vi "Main.vi"(10 "DAQ Type":enum16{"Hardware", "Simulation"}(ring), 11 "Module Admin":refnum<class "Delacor_lib_QMH_Module Admin.lvclass">) -> ()   [LabVIEW 2016, in "S-Matrix.lvlib"]
doc: "This template is based off of the Queued Message Handler design pattern and the Queued Message Handler project template that ships with LabVIEW.\n\nThe main difference is that the queue is private to this module and communication between modules is performed via Broadcast and Request events.\n\nRequest events are wrapped in public API methods and are handled in the Event Handling Loop (EHL) of this VI. Any module can register for Broadcast events sent by this module. The EHL generates messages based on user interface actions.\n\nThe Message Handling Loop (MHL) processes messages generated by the EHL, or by other messages. The messages are string values, so new messages can be added easily to the Message Cases case structure in the MHL. Each message cluster can also provide an optional value for Message Data, which is a variant that can be converted to whatever message-specific data is required.\n_____\nBased on DQMH Project Template 6.1.0.94."
uses:
  S-Matrix.lvlib
  <vilib>/Delacor/Delacor QMH/Libraries/Module Admin_class/Delacor_lib_QMH_Module Admin.lvclass
  Class/PXIe 2737/PXIe 2737.lvclass
  Class/Abstract/Abstract.lvclass
  Module Data--cluster.ctl
  Initialize Parameter.ctl
  <vilib>/Delacor/Delacor QMH/Libraries/Message Queue_class/Delacor_lib_QMH_Message Queue.lvclass/Delacor_lib_QMH_Message Queue.ctl
  Stop Argument--cluster.ctl
  <vilib>/Delacor/Delacor QMH/Libraries/Module Admin_class/Delacor_lib_QMH_Module Admin.lvclass/Delacor_lib_QMH_Module Admin.ctl
  REQ Initialize Hardware Argument--cluster.ctl
  REQ Initialize Hardware (Reply Payload)--cluster.ctl
  REQ Single Relay Argument--cluster.ctl
  REQ Close Ref Argument--cluster.ctl
  REQ Making Connection Argument--cluster.ctl
  REQ Disconnect Channel Argument--cluster.ctl
  <vilib>/Utility/miscctls.llb/LVPointTypeDef.ctl
  <vilib>/Delacor/Delacor QMH/Libraries/Message Queue_class/Delacor_lib_QMH_Enqueue Message (Single).vi
  <vilib>/Delacor/Delacor QMH/Libraries/Module Admin_class/Delacor_lib_QMH_Get External Launch.vi
  <vilib>/Utility/error.llb/Error Cluster From Error Code.vi
  <vilib>/ErrorRing/Error Ring.xnode
  <vilib>/Delacor/Delacor QMH/Libraries/Message Queue_class/Delacor_lib_QMH_Message Queue.lvclass
panel:
  out "error out":errorcluster
  out "Status":string
  in  "Simulate MHL Error":bool
  in  "Simulate EHL Error":bool
  # "Other QMH Modules communicate with this Module via its Public API (wrappers for its Request Events).\n\nThis Module communicates with other Modules via its Broadcast Events.\nAny module that wants to get these messages, just registers for this module's Broadcast events."
  # "This template is for the Delacor Modified Queued Message Handler design pattern.\n\nSee the block diagram for more information on how to use this template."
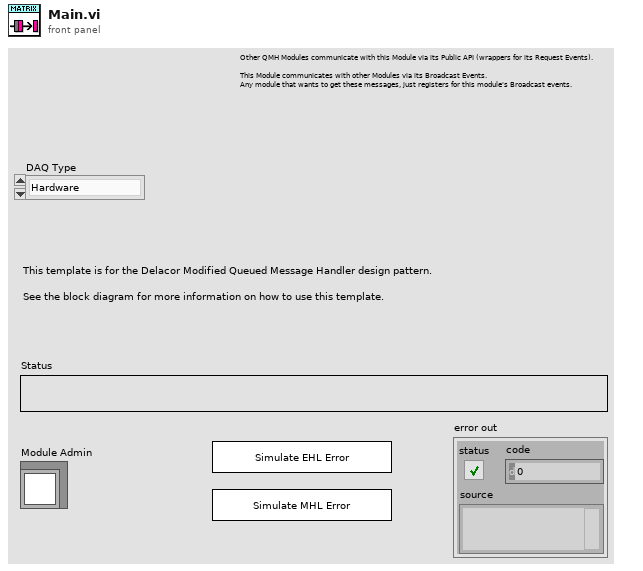
[diagram p1: front panel]
types:
  T1 = typedef "S-Matrix.lvlib/Request Events--cluster.ctl" = cluster{"Stop Module":refnum<user-event>, "Show Panel":refnum<user-event>, "Hide Panel":refnum<user-event>, "Get Module Execution Status":refnum<user-event>, "Show Diagram":refnum<user-event>, "REQ Initialize Hardware":refnum<user-event>, "REQ Single Relay":refnum<user-event>, "REQ Close Ref":refnum<user-event>, "REQ Making Connection":refnum<user-event>, "REQ Disconnect Channel":refnum<user-event>}
  T2 = typedef "S-Matrix.lvlib/Module Data--cluster.ctl" = cluster{"Status":string, "Abstract.lvclass":refnum<class "Abstract.lvclass">, "Initialize Parameter":T3}
  T3 = typedef "S-Matrix.lvlib/Initialize Parameter.ctl" = cluster{"Connection Ref":variant, "topology name":string}
  T4 = enum32{"invalid lock state", "Not Locked", "Locked (No Password)", "Password-protected"}
  T5 = typedef "S-Matrix.lvlib/Stop Argument--cluster.ctl" = cluster{"Origin":string, "Exit via Stop Module Req?":bool, "Wait for Module to stop?":bool}
  T6 = typedef "S-Matrix.lvlib/REQ Initialize Hardware Argument--cluster.ctl" = cluster{"Initialize Parameter":T3, "Wait Notifier":refnum<notifier>, "wait for reply":bool}
  T7 = typedef "S-Matrix.lvlib/REQ Single Relay Argument--cluster.ctl" = cluster{"relay name":string, "relay action":i32}
  T8 = typedef "S-Matrix.lvlib/REQ Close Ref Argument--cluster.ctl" = cluster{"Boolean":bool}
  T9 = typedef "S-Matrix.lvlib/REQ Making Connection Argument--cluster.ctl" = cluster{"First Connection":cluster{"channel 1":string, "channel 2":string}, "Second Connection":cluster{"channel 3":string, "channel 4":string}}
  T10 = typedef "S-Matrix.lvlib/REQ Disconnect Channel Argument--cluster.ctl" = cluster{"Boolean":bool}
  T11 = typedef "LVPointTypeDef.ctl" = cluster{"Horizontal":i16, "Vertical":i16}
  T12 = enum32{"Invalid", "Standard", "Closed", "Hidden", "Minimized", "Maximized"}
  T13 = typedef "S-Matrix.lvlib/REQ Initialize Hardware (Reply Payload)--cluster.ctl" = cluster{"Connect?":bool, "error":errorcluster}
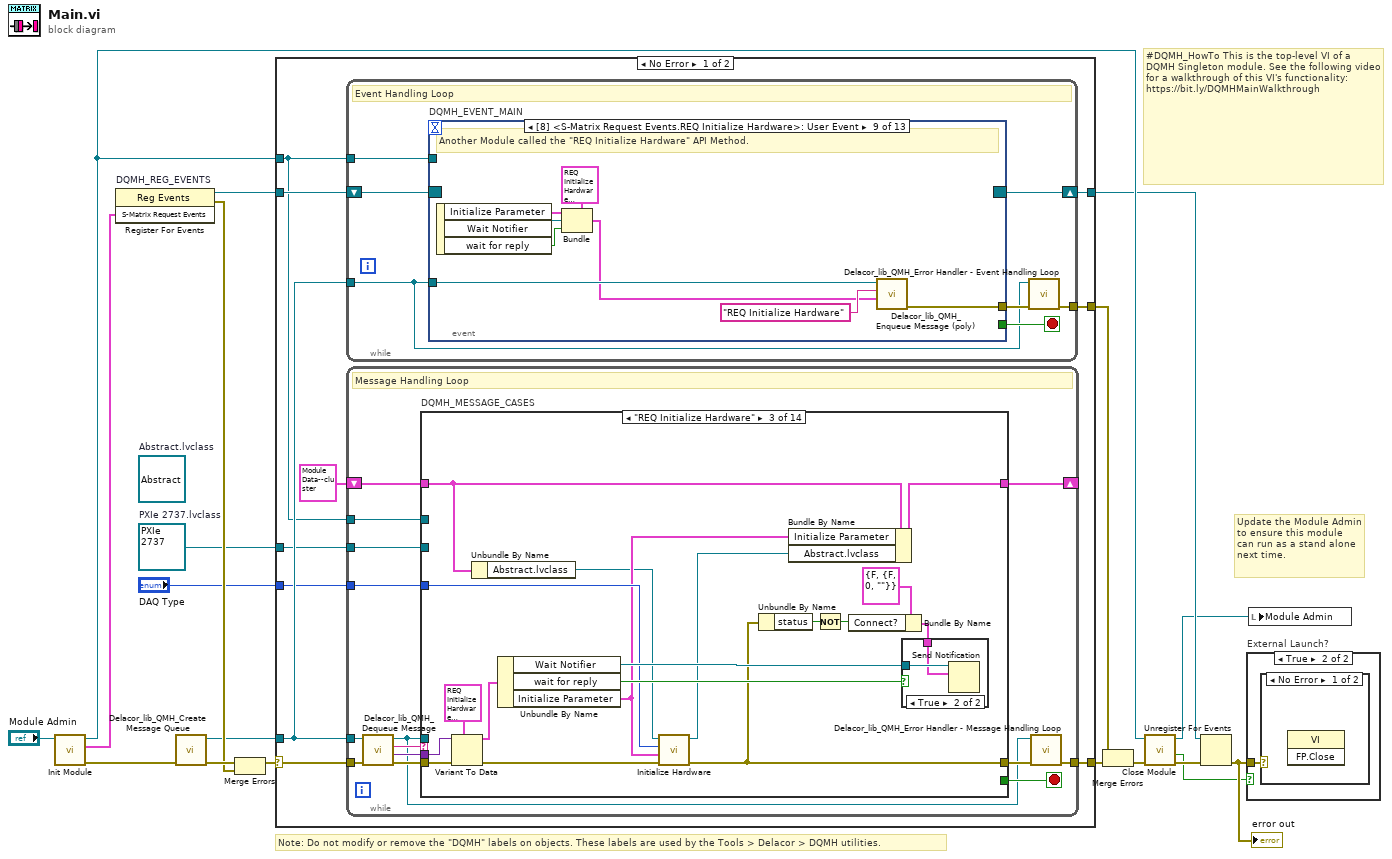
[diagram p0: block diagram]
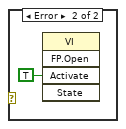
[diagram p3: hidden frame]
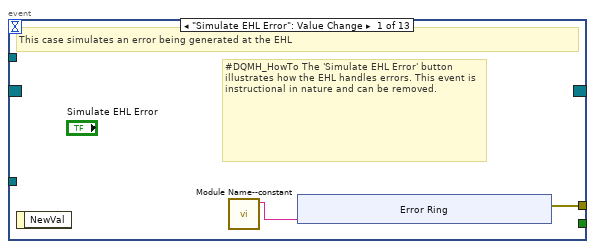
[diagram p4: hidden frame]
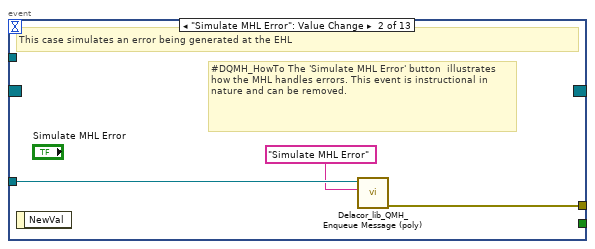
[diagram p5: hidden frame]
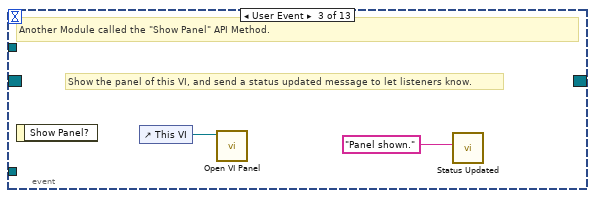
[diagram p6: hidden frame]
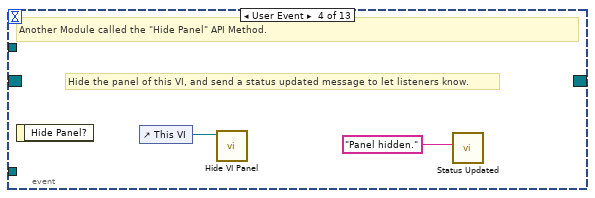
[diagram p7: hidden frame]
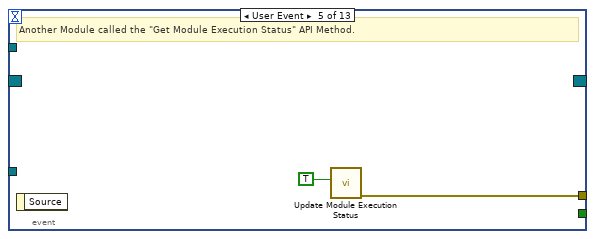
[diagram p8: hidden frame]
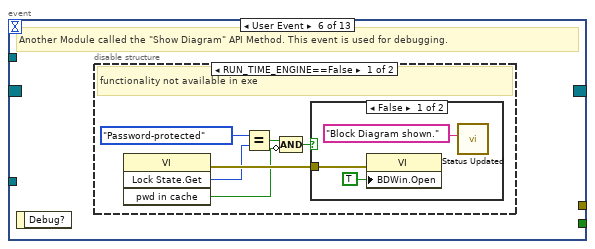
[diagram p9: hidden frame]
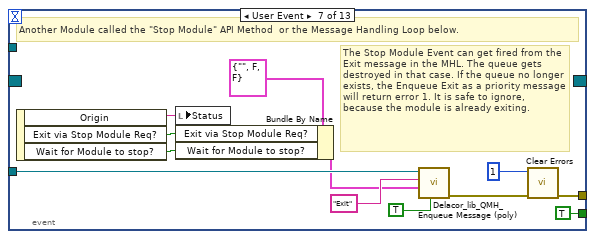
[diagram p12: hidden frame]
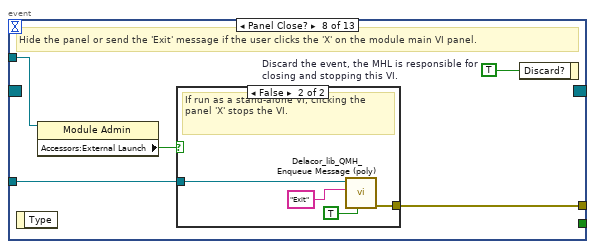
[diagram p13: hidden frame]
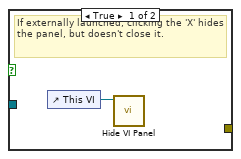
[diagram p14: hidden frame]
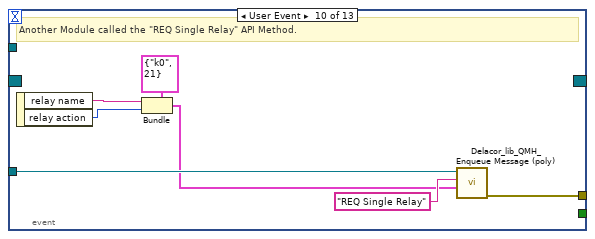
[diagram p15: hidden frame]
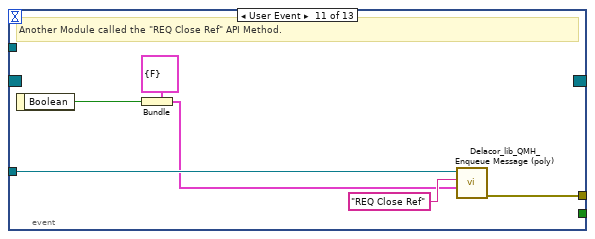
[diagram p16: hidden frame]
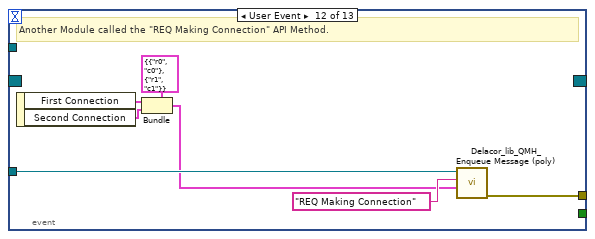
[diagram p17: hidden frame]
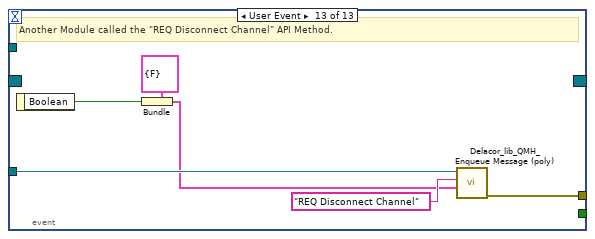
[diagram p18: hidden frame]
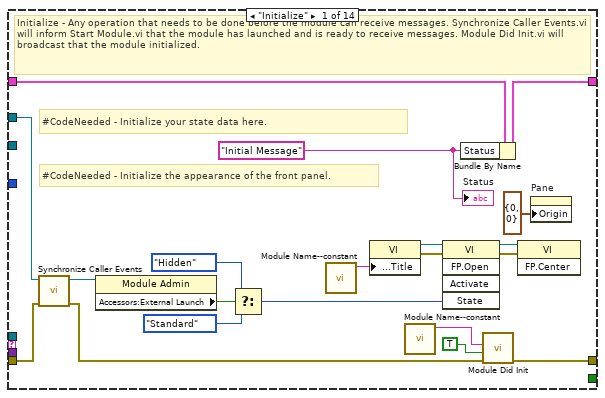
[diagram p19: hidden frame]
diagram:
  w1 = refnum<class "PXIe 2737.lvclass"> refnum  # PXIe 2737.lvclass
  (unwired) refnum<class "Abstract.lvclass"> refnum  # Abstract.lvclass
  # "#DQMH_HowTo This is the top-level VI of a DQMH Singleton module. See the following video for a walkthrough of this VI's functionality: https://bit.ly/DQMHMainWalkthrough"
  # "Note: Do not modify or remove the \"DQMH\" labels on objects. These labels are used by the Tools > Delacor > DQMH utilities."
  # "Update the Module Admin to ensure this module can run as a stand alone next time."
  n1 = call "Init Module.vi"("Singleton Module Admin in"="Module Admin") -> ("error out"=w18:errorcluster, "S-Matrix Request Events"=w7:T1, "Singleton Module Admin out"=w10:refnum<class "Delacor_lib_QMH_Module Admin.lvclass">)  [unwired: 8 in]
  n2 = register-events "DQMH_REG_EVENTS"(w7) -> (reference out=w8:refnum<event-registration>, error out=w11:errorcluster)  [unwired: 2 in]
  n3 = call <vilib>:"Delacor_lib_QMH_Create Message Queue.vi"("error in"=w18) -> ("error out"=w13:errorcluster, "Message Queue"=w6:refnum<class "Delacor_lib_QMH_Message Queue.lvclass">)  [unwired: 9 in]
  n4 = Merge Errors(w13, w11) -> (w12:errorcluster)
  n5 = case shown="No Error" w12 {
    selector: w12 -> [w27 w293]
    tunnel: [w29 w292] -> w19
    tunnel: [w26 w298] -> w9
    tunnel: w8 -> [w24 w298]
    tunnel: w6 -> [w23 w291]
    tunnel: [w28 _] -> w16
    tunnel: w10 -> [w22 w294]
    tunnel: "DAQ Type" -> [w21 _]
    tunnel: w1 -> [w20 _]
    frame No Error {
      n6 = while {
        tunnel: w23 -> [w30]
        shift-right: [w33] -> w26
        shift-left: w24 -> [w34]
        tunnel: [w35] -> w28
        tunnel: w22 -> [w31]
        stop <- w32 stop-if-true
        # "Event Handling Loop"
        n7 = event "DQMH_EVENT_MAIN" shown="[8] <S-Matrix Request Events.REQ Initialize Hardware>: User Event" {
          selector: w34 -> [_ _ _ _ _ _ _ _ _ _ _ _ _]
          dyn-events: [_ _ _ _ _ _ _ _ _ _ _ _ _] -> w33
          timeout: _ -> [_ _ _ _ _ _ _ _ _ _ _ _ _]
          tunnel: [_ _ _ _ _ _ TRUE ("Discard?") _ _ _ _ _ _] -> w32
          tunnel: w30 -> [_ w47 _ _ _ _ w71 w78 w93 w100 w106 w113 w119]
          tunnel: [w38 w48 _ _ w54 _ w74 w80 w86 w94 w101 w107 w114] -> w36
          tunnel: w31 -> [_ _ _ _ _ _ _ w77 _ _ _ _ _]
          event "Simulate EHL Error": Value Change {
            # "#DQMH_HowTo The 'Simulate EHL Error' button  illustrates how the EHL handles errors. This event is instructional in nature and can be removed."
            # "This case simulates an error being generated at the EHL"
            n8 = event-data() -> ()  [unwired: 1 in, 1 out]
            n9 = call "Module Name--constant.vi"() -> ("Module Name"=w37:string)  [unwired: 11 in]
            n10 = xnode "Error Ring"("parameter 0"=w37) -> ("error out"=w38:errorcluster)
          }
          event "Simulate MHL Error": Value Change {
            # "#DQMH_HowTo The 'Simulate MHL Error' button  illustrates how the MHL handles errors. This event is instructional in nature and can be removed."
            # "This case simulates an error being generated at the EHL"
            n11 = event-data() -> ()  [unwired: 1 in, 1 out]
            n12 = call-poly <vilib>:"Delacor_lib_QMH_Enqueue Message (poly).vi"("Message"="Simulate MHL Error", "Message Queue in"=w47) -> ("error out"=w48:errorcluster)  [unwired: 8 in, 1 out]
          }
          event User Event {
            # "Show the panel of this VI, and send a status updated message to let listeners know."
            # "Another Module called the \"Show Panel\" API Method."
            n13 = event-data() -> ()  [unwired: 1 in, 1 out]
            n14 = control-ref of="This VI"() -> (w50:refnum<vi>)
            n15 = call "Open VI Panel.vi"("VI"=w50) -> ()  [unwired: 10 in, 1 out]
            n16 = call "Status Updated.vi"("Status"="Panel shown." ("format string")) -> ()  [unwired: 10 in, 1 out]
          }
          event User Event {
            # "Hide the panel of this VI, and send a status updated message to let listeners know."
            # "Another Module called the \"Hide Panel\" API Method."
            n17 = event-data() -> ()  [unwired: 1 in, 1 out]
            n18 = control-ref of="This VI"() -> (w52:refnum<vi>)
            n19 = call "Hide VI Panel.vi"("VI"=w52) -> ()  [unwired: 10 in, 1 out]
            n20 = call "Status Updated.vi"("Status"="Panel hidden." ("format string")) -> ()  [unwired: 10 in, 1 out]
          }
          event User Event {
            # "Another Module called the \"Get Module Execution Status\" API Method."
            n21 = event-data() -> ()  [unwired: 1 in, 1 out]
            n22 = call "Update Module Execution Status.vi"("Running?"=TRUE) -> ("error out"=w54:errorcluster)  [unwired: 10 in]
          }
          event User Event {
            # "Another Module called the \"Show Diagram\" API Method. This event is used for debugging."
            n23 = event-data() -> ()  [unwired: 1 in, 1 out]
            n24 = disable-structure shown="RUN_TIME_ENGINE==False" {
              frame condition #0 (active) {
                # "functionality not available in exe"
                n25 = invoke class="VI" method="Lock State.Get"() -> (error out=w60:errorcluster, "Get Lock State"=w59:T4, "pwd in cache"=w56:bool)  [unwired: 4 in, 1 out]
                n26 = Equal?(x=T4."Password-protected", y=w59) -> (x = y?=w57:bool)
                n27 = Compound Arithmetic op=AND(w57, invert w56) -> (w55:bool)
                n28 = case shown="False" w55 {
                  tunnel: w60 -> [w63 _]
                  frame False {
                    n29 = property class="VI"(error in=w63, "BDWin.Open"=TRUE ("Block Diagram Window:Open")) -> ()  [unwired: 1 in, 2 out]
                    n30 = call "Status Updated.vi"("Status"="Block Diagram shown." ("format string")) -> ()  [unwired: 10 in, 1 out]
                  }
                  frame True {
                    # "Password-protected VI, and the password is not in the cache. Do not show the diagram."
                  }
                }
              }
              frame condition #1 {
              }
            }
          }
          event User Event {
            # "The Stop Module Event can get fired from the Exit message in the MHL. The queue gets destroyed in that case. If the queue no longer exists, the Enqueue Exit as a priority message will return error 1. It is safe to ignore, because the module is already exiting."
            # "Another Module called the \"Stop Module\" API Method  or the Message Handling Loop below."
            n31 = event-data() -> ("Origin"=w70:string, "Exit via Stop Module Req?"=w66:bool, "Wait for Module to stop?"=w65:bool)  [unwired: 1 in]
            n32 = local write "Status"(w70) -> ()
            n33 = Bundle By Name(cluster=T5 {"Origin"="", "Exit via Stop Module Req?"=FALSE, "Wait for Module to stop?"=FALSE} ("Stop Argument"), "Exit via Stop Module Req?"=w66, "Wait for Module to stop?"=w65) -> (w64:T5)
            n34 = call-poly <vilib>:"Delacor_lib_QMH_Enqueue Message (poly).vi"("Priority Message? (F)"=TRUE, "Message Data"=w64, "Message"="Exit", "Message Queue in"=w71) -> ("error out"=w75:errorcluster)  [unwired: 6 in, 1 out]
            n35 = call <vilib>:"Clear Errors.vi"("error in (no error)"=w75, "specific error code to clear (0: all)"=1) -> ("error out"=w74:errorcluster)  [unwired: 4 in, 1 out]
          }
          event Panel Close? {
            w79 = TRUE  # Discard the event, the MHL is responsible for closing and stopping this VI.
            # "Hide the panel or send the 'Exit' message if the user clicks the 'X' on the module main VI panel."
            n36 = event-data() -> ()  [unwired: 1 in, 1 out]
            n37 = property class="Module Admin"(reference=w77) -> ("Accessors:External Launch"=w76:bool)  [unwired: 1 in, 2 out]
            n38 = case shown="False" w76 {
              tunnel: w78 -> [_ w84]
              tunnel: [_ w85] -> w80
              frame True {
                # "If externally launched, clicking the 'X' hides the panel, but doesn't close it."
                n39 = control-ref of="This VI"() -> (w81:refnum<vi>)
                n40 = call "Hide VI Panel.vi"("VI"=w81) -> ()  [unwired: 10 in, 1 out]
              }
              frame False {
                # "If run as a stand-alone VI, clicking the panel 'X' stops the VI."
                n41 = call-poly <vilib>:"Delacor_lib_QMH_Enqueue Message (poly).vi"("Priority Message? (F)"=TRUE, "Message"="Exit", "Message Queue in"=w84) -> ("error out"=w85:errorcluster)  [unwired: 7 in, 1 out]
              }
            }
            n42 = event-data("Discard?"=w79) -> ()  [unwired: 1 in, 1 out]
          }
          event User Event {
            # "Another Module called the \"REQ Initialize Hardware\" API Method."
            n43 = event-data() -> ("Initialize Parameter"=w89:T3, "Wait Notifier"=w88:refnum<notifier>, "wait for reply"=w87:bool)  [unwired: 1 in]
            n44 = Bundle(cluster=T6 {"Initialize Parameter"={"Connection Ref"=variant, "topology name"="Configured Topology"}, "Wait Notifier"=refnum, "wait for reply"=FALSE} ("REQ Initialize Hardware Argument"), "Initialize Parameter"=w89, "Wait Notifier"=w88, "wait for reply"=w87) -> (w90:T6)
            n45 = call-poly <vilib>:"Delacor_lib_QMH_Enqueue Message (poly).vi"("Message Data"=w90, "Message"="REQ Initialize Hardware", "Message Queue in"=w93) -> ("error out"=w86:errorcluster)  [unwired: 7 in, 1 out]
          }
          event User Event {
            # "Another Module called the \"REQ Single Relay\" API Method."
            n46 = event-data() -> ("relay name"=w96:string, "relay action"=w95:i32)  [unwired: 1 in]
            n47 = Bundle(cluster=T7 {"relay name"="k0", "relay action"=21} ("REQ Single Relay Argument"), "relay name"=w96, "relay action"=w95) -> (w97:T7)
            n48 = call-poly <vilib>:"Delacor_lib_QMH_Enqueue Message (poly).vi"("Message Data"=w97, "Message"="REQ Single Relay", "Message Queue in"=w100) -> ("error out"=w94:errorcluster)  [unwired: 7 in, 1 out]
          }
          event User Event {
            # "Another Module called the \"REQ Close Ref\" API Method."
            n49 = event-data() -> ("Boolean"=w102:bool)  [unwired: 1 in]
            n50 = Bundle(cluster=T8 {"Boolean"=FALSE} ("REQ Close Ref Argument"), "Boolean"=w102) -> (w103:T8)
            n51 = call-poly <vilib>:"Delacor_lib_QMH_Enqueue Message (poly).vi"("Message Data"=w103, "Message"="REQ Close Ref", "Message Queue in"=w106) -> ("error out"=w101:errorcluster)  [unwired: 7 in, 1 out]
          }
          event User Event {
            # "Another Module called the \"REQ Making Connection\" API Method."
            n52 = event-data() -> ("First Connection"=w109:cluster{"channel 1":string, "channel 2":string}, "Second Connection"=w108:cluster{"channel 3":string, "channel 4":string})  [unwired: 1 in]
            n53 = Bundle(cluster=T9 {"First Connection"={"channel 1"="r0", "channel 2"="c0"}, "Second Connection"={"channel 3"="r1", "channel 4"="c1"}} ("REQ Making Connection Argument"), "First Connection"=w109, "Second Connection"=w108) -> (w110:T9)
            n54 = call-poly <vilib>:"Delacor_lib_QMH_Enqueue Message (poly).vi"("Message Data"=w110, "Message"="REQ Making Connection", "Message Queue in"=w113) -> ("error out"=w107:errorcluster)  [unwired: 7 in, 1 out]
          }
          event User Event {
            # "Another Module called the \"REQ Disconnect Channel\" API Method."
            n55 = event-data() -> ("Boolean"=w115:bool)  [unwired: 1 in]
            n56 = Bundle(cluster=T10 {"Boolean"=FALSE} ("REQ Disconnect Channel Argument"), "Boolean"=w115) -> (w116:T10)
            n57 = call-poly <vilib>:"Delacor_lib_QMH_Enqueue Message (poly).vi"("Message Data"=w116, "Message"="REQ Disconnect Channel", "Message Queue in"=w119) -> ("error out"=w114:errorcluster)  [unwired: 7 in, 1 out]
          }
        }
        n58 = call-dynamic "Delacor_lib_QMH_Error Handler - Event Handling Loop.vi"("error in"=w36, "Message Queue in"=w30) -> ("dup error in"=w35:errorcluster)  [unwired: 8 in, 1 out]
      }
      n59 = while {
        tunnel: w23 -> [w124]
        shift-right: [w128] -> _
        shift-left: T2 {"Status"="", "Abstract.lvclass"=refnum, "Initialize Parameter"={"Connection Ref"=variant, "topology name"="Configured Topology"}} ("Data Cluster") -> [w129]
        tunnel: w27 -> [w132]
        tunnel: [w130] -> w29
        tunnel: w22 -> [w122]
        tunnel: w21 -> [w121]
        tunnel: w20 -> [w120]
        stop <- w127 stop-if-true
        # "Message Handling Loop"
        n60 = call-dynamic "Delacor_lib_QMH_Dequeue Message.vi"("error in"=w132, "Message Queue in"=w124) -> ("error out"=w131:errorcluster, "Message Data"=w125:variant, "Message"=w126:string, "Message Queue out"=w123:refnum<class "Delacor_lib_QMH_Message Queue.lvclass">)  [unwired: 6 in]
        n61 = case "DQMH_MESSAGE_CASES" shown="\"REQ Initialize Hardware\"" w126 {
          selector: w126 -> [_ _ _ _ _ _ _ _ _ _ _ _ _ w278]
          tunnel: w123 -> [_ _ _ _ _ _ w215 _ _ _ _ w248 w270 _]
          tunnel: w131 -> [w151 w155 w173 w187 w199 w209 w217 w228 w231 w233 w238 w255 w276 w280]
          tunnel: [w149 w155 w162 w182 w194 w204 w216 w223 w230 w233 w237 w251 w273 w281] -> w133
          tunnel: w129 -> [w140 w154 w157 w179 w191 w203 w213 w222 w229 w232 w235 w250 w269 w279]
          tunnel: [w139 w154 w163 w177 w189 w201 w213 w220 w229 w232 w235 w250 w269 w279] -> w128
          tunnel: [_ _ _ _ _ _ _ _ _ _ _ _ w268 _] -> w127
          tunnel: w125 -> [_ _ w172 w186 w198 w208 _ w227 _ _ _ w249 w267 _]
          tunnel: w122 -> [w141 _ _ _ _ _ _ _ _ _ _ w247 w262 _]
          tunnel: w121 -> [_ _ w164 _ _ _ _ _ _ _ _ _ _ _]
          tunnel: w120 -> [_ _ _ _ _ _ _ _ _ _ _ _ _ _]
          frame "Initialize" {
            w135 = "Initial Message" ("Initial Message")
            # "#CodeNeeded - Initialize the appearance of the front panel."
            # "#CodeNeeded - Initialize your state data here."
            # "Initialize - Any operation that needs to be done before the module can receive messages. Synchronize Caller Events.vi will inform Start Module.vi that the module has launched and is ready to receive messages. Module Did Init.vi will broadcast that the module initialized."
            n62 = call "Synchronize Caller Events.vi"("error in (no error)"=w151, "Singleton Module Admin in"=w141) -> ("error out"=w150:errorcluster, "Singleton Module Admin out"=w136:refnum<class "Delacor_lib_QMH_Module Admin.lvclass">)  [unwired: 8 in]
            n63 = property class="Module Admin"(reference=w136) -> ("Accessors:External Launch"=w145:bool)  [unwired: 1 in, 2 out]
            n64 = Select(t=T12."Hidden" ("State"), s=w145, f=T12."Standard" ("State")) -> (s? t:f=w142:T12)
            n65 = call "Module Name--constant.vi"() -> ("Module Name"=w148:string)  [unwired: 11 in]
            n66 = property class="VI"("Front Panel.Title"=w148) -> (reference out=w147:refnum<vi>, error out=w153:errorcluster)  [unwired: 2 in]
            n67 = call "Module Name--constant.vi"() -> ("Module Name"=w137:string)  [unwired: 11 in]
            n68 = invoke class="VI" method="FP.Open"(reference=w147, error in=w153, "State"=w142) -> (reference out=w146:refnum<vi>, error out=w152:errorcluster)  [unwired: 2 in, 3 out]
            n69 = Bundle By Name(cluster=w140, "Status"=w135) -> (w139:T2)
            n70 = call "Module Did Init.vi"("error in (no error)"=w150, "Initialized?"=TRUE, "Origin"=w137) -> ("error out"=w149:errorcluster)  [unwired: 8 in]
            n71 = invoke class="VI" method="FP.Center"(reference=w146, error in=w152) -> ()  [unwired: 1 in, 3 out]
            n72 = property on="Pane" class="Pane"("Origin"=T11 {"Horizontal"=0, "Vertical"=0}) -> ()  [unwired: 2 in, 2 out]
            "Status" <- w135
          }
          frame "---Module Specific---" {
            # "Separator -- The following cases handle messages specific to this Module."
          }
          frame "REQ Initialize Hardware" {
            n73 = Variant To Data(error in=w173, type=T6 {"Initialize Parameter"={"Connection Ref"=variant, "topology name"="Configured Topology"}, "Wait Notifier"=refnum, "wait for reply"=FALSE} ("REQ Initialize Hardware Argument"), Variant=w172) -> (data=w170:T6, error out=w165:errorcluster)
            n74 = Unbundle By Name(w157) -> ("Abstract.lvclass"=w156:refnum<class "Abstract.lvclass">)
            n75 = Unbundle By Name(w170) -> ("Wait Notifier"=w169:refnum<notifier>, "wait for reply"=w168:bool, "Initialize Parameter"=w158:T3)
            n76 = call-dynamic "Initialize Hardware.vi"("error in (no error)"=w165, "Initialize Parameter"=w158, "DAQ Type"=w164, "Abstract in"=w156) -> ("error out"=w162:errorcluster, "Abstract out"=w159:refnum<class "Abstract.lvclass">)  [unwired: 6 in]
            n77 = Unbundle By Name(w162) -> ("status"=w161:bool)
            n78 = Bundle By Name(cluster=w157, "Initialize Parameter"=w158, "Abstract.lvclass"=w159) -> (w163:T2)
            n79 = Not(x=w161) -> (.not. x?=w160:bool)
            n80 = Bundle By Name(cluster=T13 {"Connect?"=FALSE, "error"={"status"=FALSE, "code"=0, "source"=""}} ("REQ Initialize Hardware (Reply Payload)"), "Connect?"=w160) -> (w167:T13)
            n81 = case shown="True" w168 {
              tunnel: w169 -> [_ w175]
              tunnel: w167 -> [_ w174]
              frame False {
              }
              frame True {
                n82 = Send Notification(notification=w174, notifier=w175) -> ()  [unwired: 1 in, 2 out]
              }
            }
          }
          frame "REQ Single Relay" {
            n83 = Variant To Data(error in=w187, type=T7 {"relay name"="k0", "relay action"=21} ("REQ Single Relay Argument"), Variant=w186) -> (data=w184:T7, error out=w183:errorcluster)
            n84 = Unbundle By Name(w184) -> ("relay name"=w181:string, "relay action"=w180:i32)
            n85 = Unbundle By Name(w179) -> ("Abstract.lvclass"=w178:refnum<class "Abstract.lvclass">)
            n86 = call-dynamic "Individual Relay.vi"("error in (no error)"=w183, "relay action"=w180, "relay name"=w181, "Abstract in"=w178) -> ("error out"=w182:errorcluster, "Abstract out"=w176:refnum<class "Abstract.lvclass">)  [unwired: 6 in]
            n87 = Bundle By Name(cluster=w179, "Abstract.lvclass"=w176) -> (w177:T2)
          }
          frame "REQ Making Connection" {
            n88 = Variant To Data(error in=w199, type=T9 {"First Connection"={"channel 1"="r0", "channel 2"="c0"}, "Second Connection"={"channel 3"="r1", "channel 4"="c1"}} ("REQ Making Connection Argument"), Variant=w198) -> (data=w196:T9, error out=w195:errorcluster)
            n89 = Unbundle By Name(w196) -> ("First Connection"=w193:cluster{"channel 1":string, "channel 2":string}, "Second Connection"=w192:cluster{"channel 3":string, "channel 4":string})
            n90 = Unbundle By Name(w191) -> ("Abstract.lvclass"=w190:refnum<class "Abstract.lvclass">)
            n91 = call-dynamic "Switch Making Connection.vi"("error in (no error)"=w195, "Second Connection"=w192, "First Connection"=w193, "Abstract in"=w190) -> ("error out"=w194:errorcluster, "Abstract out"=w188:refnum<class "Abstract.lvclass">)  [unwired: 6 in]
            n92 = Bundle By Name(cluster=w191, "Abstract.lvclass"=w188) -> (w189:T2)
          }
          frame "REQ Disconnect Channel" {
            n93 = Variant To Data(error in=w209, type=T10 {"Boolean"=FALSE} ("REQ Disconnect Channel Argument"), Variant=w208) -> (data=w206:T10, error out=w205:errorcluster)
            n94 = Unbundle By Name(w206) -> ()  [unwired: 1 out]
            n95 = Unbundle By Name(w203) -> ("Abstract.lvclass"=w202:refnum<class "Abstract.lvclass">)
            n96 = call-dynamic "Disconnect Channel.vi"("error in (no error)"=w205, "Abstract in"=w202) -> ("error out"=w204:errorcluster, "Abstract out"=w200:refnum<class "Abstract.lvclass">)  [unwired: 8 in]
            n97 = Bundle By Name(cluster=w203, "Abstract.lvclass"=w200) -> (w201:T2)
          }
          frame "REQ Reconnect" {
            # "Duplicate this frame when creating new messages.  Change this comment in the duplicated frame to describe this message."
            n98 = Unbundle By Name(w213) -> ("Initialize Parameter.Connection Ref"=w212:variant)
            n99 = Bundle By Name(cluster=T6 {"Initialize Parameter"={"Connection Ref"=variant, "topology name"="Configured Topology"}, "Wait Notifier"=refnum, "wait for reply"=FALSE} ("REQ Initialize Hardware Argument"), "Initialize Parameter.Connection Ref"=w212) -> (w211:T6)
            n100 = Wait (ms)(milliseconds to wait=u32 2000) -> ()  [unwired: 1 out]
            n101 = call-poly <vilib>:"Delacor_lib_QMH_Enqueue Message (poly).vi"("error in"=w217, "Message Data"=w211, "Message"="REQ Initialize Hardware", "Message Queue in"=w215) -> ("error out"=w216:errorcluster)  [unwired: 6 in, 1 out]
          }
          frame "REQ Close Ref" {
            n102 = Variant To Data(error in=w228, type=T8 {"Boolean"=FALSE} ("REQ Close Ref Argument"), Variant=w227) -> (data=w225:T8, error out=w224:errorcluster)
            n103 = Unbundle By Name(w225) -> ()  [unwired: 1 out]
            n104 = Unbundle By Name(w222) -> ("Abstract.lvclass"=w221:refnum<class "Abstract.lvclass">)
            n105 = call-dynamic "Close Ref.vi"("error in (no error)"=w224, "Abstract in"=w221) -> ("error out"=w223:errorcluster, "Abstract out"=w219:refnum<class "Abstract.lvclass">)  [unwired: 8 in]
            n106 = Bundle By Name(cluster=w222, "Abstract.lvclass"=w219) -> (w220:T2)
          }
          frame "---Copy This Frame---" {
            # "Duplicate this frame when creating new messages.  Change this comment in the duplicated frame to describe this message."
            n107 = Merge Errors(w231) -> (w230:errorcluster)
          }
          frame "---Exit and Error Handling---" {
            # "Separator - The following cases handle errors and exit messages."
          }
          frame "Simulate MHL Error" {
            # "#DQMH_HowTo The 'Simulate MHL Error' button  illustrates how the MHL handles errors. This event is instructional in nature and can be removed."
            # "Simulate an error occurring at the MHL"
            n108 = call "Module Name--constant.vi"() -> ("Module Name"=w234:string)  [unwired: 11 in]
            n109 = xnode "Error Ring"("parameter 0"=w234) -> ("error out"=w236:errorcluster)
            n110 = Merge Errors(w238, w236) -> (w237:errorcluster)
          }
          frame "Error" {
            # "#CodeRecommended - If you ever change the name of this \"Error\" message, you'll need to update the name in the Check Loop Error.vi as well."
            # "#CodeRecommended - If the module is running in standalone mode (External Launch = FALSE), this code will pop up an error dialog andcall the 'Exit' message if an error occurs. Add more fine-grained error handling here."
            # "Error - Check the error message data and respond accordingly. This message is sent by the \"Error Handler\" VIs at the end of each loop in this application."
            n111 = property class="Module Admin"(reference=w247) -> ("Accessors:External Launch"=w246:bool)  [unwired: 1 in, 2 out]
            n112 = Variant To Data(error in=w255, type=errorcluster {"status"=FALSE, "code"=0, "source"=""} ("error constant"), Variant=w249) -> (data=w256:errorcluster, error out=w253:errorcluster)
            n113 = call "Error Reported.vi"("Error"=w256) -> ()  [unwired: 10 in, 1 out]
            n114 = case shown="False" w246 {
              tunnel: [w261 _] -> w252
              tunnel: w248 -> [w259 _]
              tunnel: w256 -> [w260 _]
              frame False {
                (unwired) "Exit"
                n115 = call <vilib>:"Simple Error Handler.vi"("error in (no error)"=w260) -> ()  [unwired: 4 in, 5 out]
                n116 = call-poly <vilib>:"Delacor_lib_QMH_Enqueue Message (poly).vi"("Priority Message? (F)"=TRUE, "Message"="REQ Reconnect", "Message Queue in"=w259) -> ("error out"=w261:errorcluster)  [unwired: 7 in, 1 out]
              }
              frame True {
                # "If the module was launched externally, calling the Error Reported broadcast VI is the only action performed by the \"Error\" message. The module's caller can then process the error appropriately."
              }
            }
            n117 = Merge Errors(w253, w252) -> (w251:errorcluster)
            n118 = local write "error out"(w251) -> ()
          }
          frame "Exit" {
            w266 = 91  # 91: not all Exit messages will have an argument
            w268 = TRUE  # Stop the VI
            # "Release the message queue reference"
            # "#CodeNeeded - Add any required cleanup code here"
            # "Exit - Exit the application."
            n119 = Variant To Data(error in=w276, type=T5 {"Origin"="", "Exit via Stop Module Req?"=FALSE, "Wait for Module to stop?"=FALSE} ("Stop Argument"), Variant=w267) -> (data=w264:T5, error out=w272:errorcluster)
            n120 = call <vilib>:"Clear Errors.vi"("error in (no error)"=w272, "specific error code to clear (0: all)"=w266) -> ("error out"=w275:errorcluster)  [unwired: 4 in, 1 out]
            n121 = control-ref of="This VI"() -> (w263:refnum<vi>)
            n122 = call-dynamic "Delacor_lib_QMH_Release Message Queue.vi"("error in"=w275, "Message Queue"=w270) -> ("error out"=w274:errorcluster)  [unwired: 9 in]
            n123 = call "Handle Exit.vi"("Stop Argument"=w264, "Admin in"=w262, "VI reference"=w263) -> ("error out"=w271:errorcluster)  [unwired: 7 in, 1 out]
            n124 = Merge Errors(w274, w271) -> (w273:errorcluster)
          }
          frame Default {
            # "'Default' case only runs if there is a message that isn't defined in any of the other cases.  Output a programming error."
            n125 = call "Module Name--constant.vi"() -> ("Module Name"=w277:string)  [unwired: 11 in]
            n126 = xnode "Error Ring"("parameter 0"=w278, "parameter 1"=w277) -> ("error out"=w282:errorcluster)
            n127 = Merge Errors(w280, w282) -> (w281:errorcluster)
          }
        }
        n128 = call-dynamic "Delacor_lib_QMH_Error Handler - Message Handling Loop.vi"("error in"=w133, "Message Queue in"=w123) -> ("dup error in"=w130:errorcluster)  [unwired: 8 in, 1 out]
      }
    }
    frame Error {
      # "Synchronize Caller Events.vi will inform Start Module.vi that the module has launched and will let the code calling Start Module.vi register for broadcasts and would permit the caller receive the broadcast that an error occurred at launch time."
      n129 = call-dynamic "Delacor_lib_QMH_Release Message Queue.vi"("error in"=w293, "Message Queue"=w291) -> ("error out"=w292:errorcluster)  [unwired: 9 in]
      n130 = call "Synchronize Caller Events.vi"("Singleton Module Admin in"=w294) -> ("error out"=w299:errorcluster)  [unwired: 9 in, 1 out]
      n131 = call "Module Name--constant.vi"() -> ("Module Name"=w297:string)  [unwired: 11 in]
      n132 = Format Into String(format string="An error occurred during initialization. %s is no longer running.", w297) -> (resulting string=w295:string)  [unwired: 2 in, 1 out]
      n133 = Merge Errors(w292, w299) -> (w300:errorcluster)
      n134 = call "Error Reported.vi"("Additional Information"=w295, "Error"=w300) -> ()  [unwired: 9 in, 1 out]
    }
  }
  n135 = Merge Errors(w16, w19) -> (w15:errorcluster)
  n136 = call "Close Module.vi"("error in (no error)"=w15, "Module Admin in"=w10) -> ("error out"=w17:errorcluster, "External Launch"=w3:bool, "Module Admin out"=w4:refnum<class "Delacor_lib_QMH_Module Admin.lvclass">)  [unwired: 7 in]
  n137 = Unregister For Events(event registration refnum=w9, error in=w17) -> (error out=w14:errorcluster)
  "error out" <- w14
  n138 = case "External Launch?" shown="True" w3 {
    tunnel: w14 -> [_ w301]
    frame False {
    }
    frame True {
      n139 = case shown="No Error" w301 {
        frame No Error {
          n140 = invoke class="VI" method="FP.Close"() -> ()  [unwired: 3 in, 3 out]
        }
        frame Error {
          n141 = invoke class="VI" method="FP.Open"("Activate"=TRUE ("Activate?")) -> ()  [unwired: 4 in, 5 out]
        }
      }
    }
  }
  n142 = local write "Module Admin"(w4) -> ()
